vi "SaveStriptestRecoveryFiles.vi"(3 "Array Titles":string, 4 "Strip Segment":string, 7 "Region #":u32) -> (0 "Path + Filename OUT":string, 1 "Filename OUT":string)   [LabVIEW 2018]
uses:
  general_VIs/globals/QC_RunInformation.vi
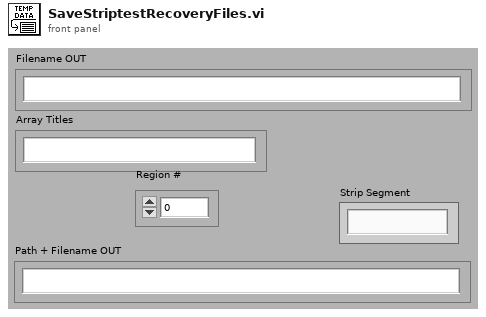
[diagram p1: front panel]
types:
  T1 = enum16{"open", "open or create", "create or replace", "create"}
  T2 = cluster{"Institute":string, "Manufacturers":string[], "Devices":string[], "Serialnumbers Lookup DB":string, "Data directory":string, "Backup & screenshot directory":string, "List of known users":string[], "Measurement switch not used":bool, "Measurement Switch":string, "DUT Switch":string, "Rseries IV [MOhm]":string, "Rshunt IV [MOhm]":string, "Rseries CV [MOhm]":string, "DC blocking Cap [µF]":string, "Rseries LCR [MOhm]":string, "Rseries stability [MOhm]":string, "Rshunt stability [MOhm]":string, "Rseries striptest bias [MOhm]":string, "Rseries strip pinhole [MOhm]":string}
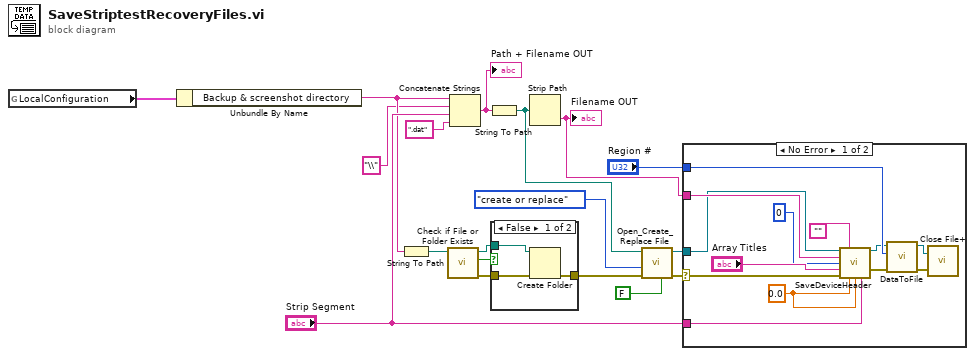
[diagram p0: block diagram]
diagram:
  n1 = global read "QC_RunInformation.vi" "LocalConfiguration"() -> (w10:T2)
  n2 = Unbundle By Name(w10) -> ("Backup & screenshot directory"=w3:string)
  n3 = String To Path(string=w3) -> (path=w4:path)
  n4 = call <vilib>:"Check if File or Folder Exists.vi"("path"=w4) -> ("error out"=w7:errorcluster, "file or folder exists?"=w6:bool, "dup path"=w5:path)  [unwired: 8 in]
  n5 = Concatenate Strings(w3, "\\" ("Substring"), "Strip Segment", ".dat") -> (w12:string)
  "Path + Filename OUT" <- w12
  n6 = String To Path(string=w12) -> (path=w15:path)
  n7 = case shown="False" w6 {
    tunnel: [w21 w22] -> w2
    tunnel: w5 -> [w20 _]
    tunnel: w7 -> [w19 w22]
    frame False {
      n8 = Create Folder(path (use dialog)=w20, error in=w19) -> (error out=w21:errorcluster)  [unwired: 1 in, 2 out]
    }
    frame True {
    }
  }
  n9 = Strip Path(path=w15) -> (name=w16:string)  [unwired: 1 out]
  "Filename OUT" <- w16
  n10 = call <vilib>:"Open_Create_Replace File.vi"("advisory dialog? (display:T)"=FALSE, "error in (no error)"=w2, "function (open:0)"=T1."create or replace", "file path"=w15) -> ("error out"=w14:errorcluster, "refnum"=w17:refnum<file>)  [unwired: 4 in, 2 out]
  n11 = case shown="No Error" w14 {
    selector: w14 -> [w35 _]
    tunnel: w17 -> [w32 _]
    tunnel: w16 -> [w33 _]
    tunnel: "Region #" -> [w28 _]
    tunnel: "Strip Segment" -> [w31 _]
    frame No Error {
      w23 = 0.0
      n12 = call "SaveDeviceHeader.vi"("File Refnum in"=w32, "no. of arrays"="", "Filename"=w33, "Run Number"=0, "Array Titles"="Array Titles", "error in (no error)"=w35, "Temperature"=w23, "Humidity"=w23, "Strip Segment"=w31) -> ("File Refnum out"=w26:refnum<file>, "error out"=w27:errorcluster)  [unwired: 4 in, 1 out]
      n13 = call "DataToFile.vi"("error in (no error)"=w27, "Sensor Index/\nSegment No."=w28, "File Refnum in"=w26) -> ("error out"=w24:errorcluster, "File Refnum out"=w25:refnum<file>)  [unwired: 7 in]
      n14 = call <vilib>:"Close File+.vi"("error in (no error)"=w24, "refnum"=w25) -> ()  [unwired: 3 in, 3 out]
    }
    frame Error {
    }
  }
